vi "FeedbackDecode_BuildMSMSSphere.vi"(4 "CompArray":T2(array[cluster])=[{"Name"="\"LittleSphereJ\"", "Type"="\"Trans3Joint\"", "ID"="J", "Num"="86", "COM"=[], "Offset"=[], "RotationAxis"=[], "OrientationMatrix"=[[1.0, 0.0, 0.0], [0.0, 1.0, 0.0], [0.0, 0.0, 1.0]], "MinAngle"=nan, "MaxAngle"=nan, "InboardID"="S", "InboardNum"="1110", "InboardCOM"=[0.0, 0.0, 0.0], "OutboardID"="S", "OutboardNum"="84", "OutboardCOM"=[0.0, 0.0, 0.0]}, {"Name"="\"IndexSphereJ\"", "Type"="\"Trans3Joint\"", "ID"="J", "Num"="94", "COM"=[], "Offset"=[], "RotationAxis"=[], "OrientationMatrix"=[[1.0, 0.0, 0.0], [0.0, 1.0, 0.0], [0.0, 0.0, 1.0]], "MinAngle"=nan, "MaxAngle"=nan, "InboardID"="S", "InboardNum"="1110", "InboardCOM"=[0.0, 0.0, 0.0], "OutboardID"="S", "OutboardNum"="92", "OutboardCOM"=[0.0, 0.0, 0.0]}, {"Name"="\"LittleKnuckle\"", "Type"="\"PinJoint\"", "ID"="J", "Num"="1160", "COM"=[], "Offset"=[], "RotationAxis"=[-0.982409, 0.0686967, 0.173648], "OrientationMatrix"=[[1.0, 0.0, 0.0], [0.0, 1.0, 0.0], [0.0, 0.0, 1.0]], "MinAngle"=0.0, "MaxAngle"=3.140021857262998, "InboardID"="S", "InboardNum"="1122", "InboardCOM"=[-0.01026417, -0.01431899999999997, 0.005183300000000002], "OutboardID"="S", "OutboardNum"="112", "OutboardCOM"=[0.0, 0.0, 0.0]}, {"Name"="\"LittleSide\"", "Type"="\"PinJoint\"", "ID"="J", "Num"="1161", "COM"=[], "Offset"=[], "RotationAxis"=[0.173225, -0.0121131, -0.984808], "OrientationMatrix"=[[1.0, 0.0, 0.0], [0.0, 1.0, 0.0], [0.0, 0.0, 1.0]], "MinAngle"=0.0, "MaxAngle"=3.140021857262998, "InboardID"="S", "InboardNum"="1110", "InboardCOM"=[-0.02813713, -0.080592, -0.0049779], "OutboardID"="S", "OutboardNum"="1122", "OutboardCOM"=[0.0, 0.0, 0.0]}, {"Name"="\"RingPIP\"", "Type"="\"PinJoint\"", "ID"="J", "Num"="1162", "COM"=[], "Offset"=[], "RotationAxis"=[-0.993768, 0.069491, 0.0871557], "OrientationMatrix"=[[1.0, 0.0, 0.0], [0.0, 1.0, 0.0], [0.0, 0.0, 1.0]], "MinAngle"=0.0, "MaxAngle"=3.140021857262998, "InboardID"="S", "InboardNum"="1125", "InboardCOM"=[-0.00263497, -0.03339700000000001, 2.619999999999706e-05], "OutboardID"="S", "OutboardNum"="1121", "OutboardCOM"=[0.0, 0.0, 0.0]}, {"Name"="\"ThumbKnuckle\"", "Type"="\"PinJoint\"", "ID"="J", "Num"="1163", "COM"=[], "Offset"=[], "RotationAxis"=[-0.130028, -0.197163, -0.97171], "OrientationMatrix"=[[1.0, 0.0, 0.0], [0.0, 1.0, 0.0], [0.0, 0.0, 1.0]], "MinAngle"=0.0, "MaxAngle"=3.140021857262998, "InboardID"="S", "InboardNum"="1113", "InboardCOM"=[0.0221366, -0.0038129999999999553, 0.00214783], "OutboardID"="S", "OutboardNum"="111", "OutboardCOM"=[0.0, 0.0, 0.0]}, {"Name"="\"RingSide\"", "Type"="\"PinJoint\"", "ID"="J", "Num"="1164", "COM"=[], "Offset"=[], "RotationAxis"=[0.0869434, -0.00607968, -0.996195], "OrientationMatrix"=[[1.0, 0.0, 0.0], [0.0, 1.0, 0.0], [0.0, 0.0, 1.0]], "MinAngle"=0.0, "MaxAngle"=3.140021857262998, "InboardID"="S", "InboardNum"="1110", "InboardCOM"=[-0.0087988, -0.08356699999999995, -0.008058199999999998], "OutboardID"="S", "OutboardNum"="1123", "OutboardCOM"=[0.0, 0.0, 0.0]}, {"Name"="\"RingKnuckle\"", "Type"="\"PinJoint\"", "ID"="J", "Num"="1165", "COM"=[], "Offset"=[], "RotationAxis"=[-0.993768, 0.069491, 0.0871557], "OrientationMatrix"=[[1.0, 0.0, 0.0], [0.0, 1.0, 0.0], [0.0, 0.0, 1.0]], "MinAngle"=0.0, "MaxAngle"=3.140021857262998, "InboardID"="S", "InboardNum"="1123", "InboardCOM"=[-0.01067969, -0.014290000000000025, 0.0043582], "OutboardID"="S", "OutboardNum"="1125", "OutboardCOM"=[0.0, 0.0, 0.0]}, {"Name"="\"ShoulderRoll\"", "Type"="\"PinJoint\"", "ID"="J", "Num"="1166", "COM"=[], "Offset"=[], "RotationAxis"=[0.0, -1.0, 0.0], "OrientationMatrix"=[[1.0, 0.0, 0.0], [0.0, 1.0, 0.0], [0.0, 0.0, 1.0]], "MinAngle"=0.0, "MaxAngle"=3.140021857262998, "InboardID"="S", "InboardNum"="1127", "InboardCOM"=[0.0346, -0.26093099999999997, 0.0], "OutboardID"="S", "OutboardNum"="116", "OutboardCOM"=[0.0, 0.0, 0.0]}, {"Name"="\"MiddleDIP\"", "Type"="\"PinJoint\"", "ID"="J", "Num"="1167", "COM"=[], "Offset"=[], "RotationAxis"=[-1.0, 0.0, 0.0], "OrientationMatrix"=[[1.0, 0.0, 0.0], [0.0, 1.0, 0.0], [0.0, 0.0, 1.0]], "MinAngle"=0.0, "MaxAngle"=3.14, "InboardID"="S", "InboardNum"="113", "InboardCOM"=[0.0197, -0.022077000000000013, -0.0010000000000000009], "OutboardID"="S", "OutboardNum"="1114", "OutboardCOM"=[0.0, 0.0, 0.0]}, {"Name"="\"IndexDIP\"", "Type"="\"PinJoint\"", "ID"="J", "Num"="1168", "COM"=[], "Offset"=[], "RotationAxis"=[-1.0, 0.0, 0.0], "OrientationMatrix"=[[1.0, 0.0, 0.0], [0.0, 1.0, 0.0], [0.0, 0.0, 1.0]], "MinAngle"=0.0, "MaxAngle"=3.140021857262998, "InboardID"="S", "InboardNum"="1124", "InboardCOM"=[0.019699999999999995, -0.017971999999999988, -0.0009999999999999974], "OutboardID"="S", "OutboardNum"="1117", "OutboardCOM"=[0.0, 0.0, 0.0]}, {"Name"="\"IndexKnuckle\"", "Type"="\"PinJoint\"", "ID"="J", "Num"="1169", "COM"=[], "Offset"=[], "RotationAxis"=[-1.0, 0.0, 0.0], "OrientationMatrix"=[[1.0, 0.0, 0.0], [0.0, 1.0, 0.0], [0.0, 0.0, 1.0]], "MinAngle"=0.0, "MaxAngle"=3.140021857262998, "InboardID"="S", "InboardNum"="1118", "InboardCOM"=[-0.0071716, -0.017827999999999955, 0.0025407999999999993], "OutboardID"="S", "OutboardNum"="1126", "OutboardCOM"=[0.0, 0.0, 0.0]}, {"Name"="\"MiddleKnuckle\"", "Type"="\"PinJoint\"", "ID"="J", "Num"="1170", "COM"=[], "Offset"=[], "RotationAxis"=[-1.0, 0.0, 0.0], "OrientationMatrix"=[[1.0, 0.0, 0.0], [0.0, 1.0, 0.0], [0.0, 0.0, 1.0]], "MinAngle"=0.0, "MaxAngle"=3.140021857262998, "InboardID"="S", "InboardNum"="1110", "InboardCOM"=[-0.00031180000000000097, -0.09855000000000003, -0.0048641], "OutboardID"="S", "OutboardNum"="1119", "OutboardCOM"=[0.0, 0.0, 0.0]}, {"Name"="\"RingSphereJ\"", "Type"="\"Trans3Joint\"", "ID"="J", "Num"="15", "COM"=[], "Offset"=[], "RotationAxis"=[], "OrientationMatrix"=[[1.0, 0.0, 0.0], [0.0, 1.0, 0.0], [0.0, 0.0, 1.0]], "MinAngle"=nan, "MaxAngle"=nan, "InboardID"="S", "InboardNum"="1110", "InboardCOM"=[0.0, 0.0, 0.0], "OutboardID"="S", "OutboardNum"="18", "OutboardCOM"=[0.0, 0.0, 0.0]}, {"Name"="\"MiddleSphereJ\"", "Type"="\"Trans3Joint\"", "ID"="J", "Num"="11", "COM"=[], "Offset"=[], "RotationAxis"=[], "OrientationMatrix"=[[1.0, 0.0, 0.0], [0.0, 1.0, 0.0], [0.0, 0.0, 1.0]], "MinAngle"=nan, "MaxAngle"=nan, "InboardID"="S", "InboardNum"="1110", "InboardCOM"=[0.0, 0.0, 0.0], "OutboardID"="S", "OutboardNum"="14", "OutboardCOM"=[0.0, 0.0, 0.0]}, {"Name"="\"ThumbSphereJ\"", "Type"="\"Trans3Joint\"", "ID"="J", "Num"="23", "COM"=[], "Offset"=[], "RotationAxis"=[], "OrientationMatrix"=[[1.0, 0.0, 0.0], [0.0, 1.0, 0.0], [0.0, 0.0, 1.0]], "MinAngle"=nan, "MaxAngle"=nan, "InboardID"="S", "InboardNum"="1110", "InboardCOM"=[0.0, 0.0, 0.0], "OutboardID"="S", "OutboardNum"="22", "OutboardCOM"=[0.0, 0.0, 0.0]}, {"Name"="\"RingDIP\"", "Type"="\"PinJoint\"", "ID"="J", "Num"="1144", "COM"=[], "Offset"=[], "RotationAxis"=[-0.993768, 0.069491, 0.0871557], "OrientationMatrix"=[[1.0, 0.0, 0.0], [0.0, 1.0, 0.0], [0.0, 0.0, 1.0]], "MinAngle"=0.0, "MaxAngle"=3.140021857262998, "InboardID"="S", "InboardNum"="1121", "InboardCOM"=[0.01818386, -0.020046000000000008, -0.002713199999999999], "OutboardID"="S", "OutboardNum"="115", "OutboardCOM"=[0.0, 0.0, 0.0]}, {"Name"="\"ElbowPitch\"", "Type"="\"PinJoint\"", "ID"="J", "Num"="1145", "COM"=[], "Offset"=[], "RotationAxis"=[0.0, 0.0, 1.0], "OrientationMatrix"=[[1.0, 0.0, 0.0], [0.0, 1.0, 0.0], [0.0, 0.0, 1.0]], "MinAngle"=0.0, "MaxAngle"=3.140021857262998, "InboardID"="S", "InboardNum"="116", "InboardCOM"=[0.019, -0.013836000000000015, -0.009000000000000001], "OutboardID"="S", "OutboardNum"="1111", "OutboardCOM"=[0.0, 0.0, 0.0]}, {"Name"="\"WristPitch\"", "Type"="\"PinJoint\"", "ID"="J", "Num"="1146", "COM"=[], "Offset"=[], "RotationAxis"=[-1.0, 0.0, 0.0], "OrientationMatrix"=[[1.0, 0.0, 0.0], [0.0, 1.0, 0.0], [0.0, 0.0, 1.0]], "MinAngle"=-0.7853981633974483, "MaxAngle"=0.7853981633974483, "InboardID"="S", "InboardNum"="114", "InboardCOM"=[0.042499999999999996, -0.16914000000000007, 0.0], "OutboardID"="S", "OutboardNum"="119", "OutboardCOM"=[0.0, 0.0, 0.0]}, {"Name"="\"ThumbDIP\"", "Type"="\"PinJoint\"", "ID"="J", "Num"="1147", "COM"=[], "Offset"=[], "RotationAxis"=[-0.130028, -0.197163, -0.97171], "OrientationMatrix"=[[1.0, 0.0, 0.0], [0.0, 1.0, 0.0], [0.0, 0.0, 1.0]], "MinAngle"=0.0, "MaxAngle"=3.14, "InboardID"="S", "InboardNum"="111", "InboardCOM"=[0.018637, -0.022448000000000023, -0.01061123], "OutboardID"="S", "OutboardNum"="1116", "OutboardCOM"=[0.0, 0.0, 0.0]}, {"Name"="\"IndexSide\"", "Type"="\"PinJoint\"", "ID"="J", "Num"="1148", "COM"=[], "Offset"=[], "RotationAxis"=[0.0, 0.0, -1.0], "OrientationMatrix"=[[1.0, 0.0, 0.0], [0.0, 1.0, 0.0], [0.0, 0.0, 1.0]], "MinAngle"=0.0, "MaxAngle"=3.140021857262998, "InboardID"="S", "InboardNum"="1110", "InboardCOM"=[0.027229700000000003, -0.07779400000000003, -0.0051141], "OutboardID"="S", "OutboardNum"="1118", "OutboardCOM"=[0.0, 0.0, 0.0]}, {"Name"="\"MiddlePIP\"", "Type"="\"PinJoint\"", "ID"="J", "Num"="1149", "COM"=[], "Offset"=[], "RotationAxis"=[-1.0, 0.0, 0.0], "OrientationMatrix"=[[1.0, 0.0, 0.0], [0.0, 1.0, 0.0], [0.0, 0.0, 1.0]], "MinAngle"=0.0, "MaxAngle"=3.140021857262998, "InboardID"="S", "InboardNum"="1119", "InboardCOM"=[-0.0002999999999999982, -0.0383, 0.0], "OutboardID"="S", "OutboardNum"="113", "OutboardCOM"=[0.0, 0.0, 0.0]}, {"Name"="\"ShoulderYaw\"", "Type"="\"PinJoint\"", "ID"="J", "Num"="1150", "COM"=[], "Offset"=[], "RotationAxis"=[0.0, 0.0, 1.0], "OrientationMatrix"=[[1.0, 0.0, 0.0], [0.0, 1.0, 0.0], [0.0, 0.0, 1.0]], "MinAngle"=0.0, "MaxAngle"=3.140021857262998, "InboardID"="S", "InboardNum"="117", "InboardCOM"=[-1.45121e-10, 0.000384746, -0.003098433], "OutboardID"="S", "OutboardNum"="1120", "OutboardCOM"=[0.0, 0.0, 0.0]}, {"Name"="\"ThumbSide\"", "Type"="\"PinJoint\"", "ID"="J", "Num"="1151", "COM"=[], "Offset"=[], "RotationAxis"=[0.691978, 0.683845, -0.23135], "OrientationMatrix"=[[1.0, 0.0, 0.0], [0.0, 1.0, 0.0], [0.0, 0.0, 1.0]], "MinAngle"=-0.7853981633974483, "MaxAngle"=0.7853981633974483, "InboardID"="S", "InboardNum"="118", "InboardCOM"=[0.008416800000000002, -0.028861000000000026, 0.0017169000000000004], "OutboardID"="S", "OutboardNum"="1113", "OutboardCOM"=[0.0, 0.0, 0.0]}, {"Name"="\"LittleDIP\"", "Type"="\"PinJoint\"", "ID"="J", "Num"="1152", "COM"=[], "Offset"=[], "RotationAxis"=[-0.982409, 0.0686967, 0.173648], "OrientationMatrix"=[[1.0, 0.0, 0.0], [0.0, 1.0, 0.0], [0.0, 0.0, 1.0]], "MinAngle"=0.0, "MaxAngle"=3.140021857262998, "InboardID"="S", "InboardNum"="1115", "InboardCOM"=[0.01887955, -0.014112000000000013, -0.004509900000000001], "OutboardID"="S", "OutboardNum"="1112", "OutboardCOM"=[0.0, 0.0, 0.0]}, {"Name"="\"WristYaw\"", "Type"="\"PinJoint\"", "ID"="J", "Num"="1153", "COM"=[], "Offset"=[], "RotationAxis"=[0.0, 0.0, -1.0], "OrientationMatrix"=[[1.0, 0.0, 0.0], [0.0, 1.0, 0.0], [0.0, 0.0, 1.0]], "MinAngle"=-0.7853981633974483, "MaxAngle"=0.7853981633974483, "InboardID"="S", "InboardNum"="119", "InboardCOM"=[-0.0425218, -0.006901999999999964, -0.004796100000000001], "OutboardID"="S", "OutboardNum"="1110", "OutboardCOM"=[0.0, 0.0, 0.0]}, {"Name"="\"IndexPIP\"", "Type"="\"PinJoint\"", "ID"="J", "Num"="1154", "COM"=[], "Offset"=[], "RotationAxis"=[-1.0, 0.0, 0.0], "OrientationMatrix"=[[1.0, 0.0, 0.0], [0.0, 1.0, 0.0], [0.0, 0.0, 1.0]], "MinAngle"=0.0, "MaxAngle"=3.140021857262998, "InboardID"="S", "InboardNum"="1126", "InboardCOM"=[-0.00030000000000000165, -0.03400000000000003, 0.0], "OutboardID"="S", "OutboardNum"="1124", "OutboardCOM"=[0.0, 0.0, 0.0]}, {"Name"="\"LittlePIP\"", "Type"="\"PinJoint\"", "ID"="J", "Num"="1155", "COM"=[], "Offset"=[], "RotationAxis"=[-0.982409, 0.0686967, 0.173648], "OrientationMatrix"=[[1.0, 0.0, 0.0], [0.0, 1.0, 0.0], [0.0, 0.0, 1.0]], "MinAngle"=0.0, "MaxAngle"=3.140021857262998, "InboardID"="S", "InboardNum"="112", "InboardCOM"=[-0.0021084, -0.02591600000000005, 5.209999999999937e-05], "OutboardID"="S", "OutboardNum"="1115", "OutboardCOM"=[0.0, 0.0, 0.0]}, {"Name"="\"ThumbMeta\"", "Type"="\"PinJoint\"", "ID"="J", "Num"="1156", "COM"=[], "Offset"=[], "RotationAxis"=[-0.0212682, -0.997909, -0.0610298], "OrientationMatrix"=[[1.0, 0.0, 0.0], [0.0, 1.0, 0.0], [0.0, 0.0, 1.0]], "MinAngle"=0.0, "MaxAngle"=3.14, "InboardID"="S", "InboardNum"="1110", "InboardCOM"=[0.015011799999999999, -0.011859999999999982, 0.0126182], "OutboardID"="S", "OutboardNum"="118", "OutboardCOM"=[0.0, 0.0, 0.0]}, {"Name"="\"ShoulderOblique\"", "Type"="\"PinJoint\"", "ID"="J", "Num"="1157", "COM"=[], "Offset"=[], "RotationAxis"=[0.57735, 0.57735, 0.57735], "OrientationMatrix"=[[1.0, 0.0, 0.0], [0.0, 1.0, 0.0], [0.0, 0.0, 1.0]], "MinAngle"=0.0, "MaxAngle"=3.14, "InboardID"="S", "InboardNum"="12", "InboardCOM"=[-0.09, -0.05, -0.26], "OutboardID"="S", "OutboardNum"="117", "OutboardCOM"=[0.0, 0.0, 0.0]}, {"Name"="\"ShoulderPitch\"", "Type"="\"PinJoint\"", "ID"="J", "Num"="1158", "COM"=[], "Offset"=[], "RotationAxis"=[-1.0, 0.0, 0.0], "OrientationMatrix"=[[1.0, 0.0, 0.0], [0.0, 1.0, 0.0], [0.0, 0.0, 1.0]], "MinAngle"=0.0, "MaxAngle"=3.140021857262998, "InboardID"="S", "InboardNum"="1120", "InboardCOM"=[-0.0346, -0.005, -0.0125], "OutboardID"="S", "OutboardNum"="1127", "OutboardCOM"=[0.0, 0.0, 0.0]}, {"Name"="\"WristRoll\"", "Type"="\"PinJoint\"", "ID"="J", "Num"="1159", "COM"=[], "Offset"=[], "RotationAxis"=[0.0, -1.0, 0.0], "OrientationMatrix"=[[1.0, 0.0, 0.0], [0.0, 1.0, 0.0], [0.0, 0.0, 1.0]], "MinAngle"=-1.5707963267948966, "MaxAngle"=1.5707963267948966, "InboardID"="S", "InboardNum"="1111", "InboardCOM"=[0.0, -0.06298999999999999, 0.003020000000000002], "OutboardID"="S", "OutboardNum"="114", "OutboardCOM"=[0.0, 0.0, 0.0]}, {"Name"="\"WristSphereJ\"", "Type"="\"Trans3Joint\"", "ID"="J", "Num"="88", "COM"=[], "Offset"=[], "RotationAxis"=[], "OrientationMatrix"=[[1.0, 0.0, 0.0], [0.0, 1.0, 0.0], [0.0, 0.0, 1.0]], "MinAngle"=nan, "MaxAngle"=nan, "InboardID"="S", "InboardNum"="114", "InboardCOM"=[0.0, 0.0, 0.0], "OutboardID"="S", "OutboardNum"="87", "OutboardCOM"=[0.0, 0.0, 0.0]}, {"Name"="\"LittleSphere\"", "Type"="\"Segment\"", "ID"="S", "Num"="84", "COM"=[0.0, 0.0, 0.0], "Offset"=[0.0, 0.0, 0.0], "RotationAxis"=[], "OrientationMatrix"=[], "MinAngle"=nan, "MaxAngle"=nan, "InboardID"="", "InboardNum"="", "InboardCOM"=[], "OutboardID"="", "OutboardNum"="", "OutboardCOM"=[]}, {"Name"="\"IndexSphere\"", "Type"="\"Segment\"", "ID"="S", "Num"="92", "COM"=[0.0, 0.0, 0.0], "Offset"=[0.0, 0.0, 0.0], "RotationAxis"=[], "OrientationMatrix"=[], "MinAngle"=nan, "MaxAngle"=nan, "InboardID"="", "InboardNum"="", "InboardCOM"=[], "OutboardID"="", "OutboardNum"="", "OutboardCOM"=[]}, {"Name"="\"ShoulderHR\"", "Type"="\"Segment\"", "ID"="S", "Num"="1127", "COM"=[0.03942751, -0.096221, -2.3999999999996247e-06], "Offset"=[0.0346, 0.005, 0.01541], "RotationAxis"=[], "OrientationMatrix"=[], "MinAngle"=nan, "MaxAngle"=nan, "InboardID"="", "InboardNum"="", "InboardCOM"=[], "OutboardID"="", "OutboardNum"="", "OutboardCOM"=[]}, {"Name"="\"ThumbProximal\"", "Type"="\"Segment\"", "ID"="S", "Num"="111", "COM"=[0.010053400000000004, -0.01129800000000003, -0.003517029999999999], "Offset"=[-0.0645434, 0.563333, 0.00970317], "RotationAxis"=[], "OrientationMatrix"=[], "MinAngle"=nan, "MaxAngle"=nan, "InboardID"="", "InboardNum"="", "InboardCOM"=[], "OutboardID"="", "OutboardNum"="", "OutboardCOM"=[]}, {"Name"="\"LittleProximal\"", "Type"="\"Segment\"", "ID"="S", "Num"="112", "COM"=[0.0086144, -0.013174000000000019, -0.0019825000000000016], "Offset"=[0.0194231, 0.61371, 0.0259807], "RotationAxis"=[], "OrientationMatrix"=[], "MinAngle"=nan, "MaxAngle"=nan, "InboardID"="", "InboardNum"="", "InboardCOM"=[], "OutboardID"="", "OutboardNum"="", "OutboardCOM"=[]}, {"Name"="\"MiddleMedial\"", "Type"="\"Segment\"", "ID"="S", "Num"="113", "COM"=[0.009050299999999997, -0.011116000000000015, -0.0009771999999999975], "Offset"=[-0.0183664, 0.655649, 0.0310502], "RotationAxis"=[], "OrientationMatrix"=[], "MinAngle"=nan, "MaxAngle"=nan, "InboardID"="", "InboardNum"="", "InboardCOM"=[], "OutboardID"="", "OutboardNum"="", "OutboardCOM"=[]}, {"Name"="\"Forearm\"", "Type"="\"Segment\"", "ID"="S", "Num"="114", "COM"=[-1.860000000000056e-05, -0.08232500000000004, -9.750000000000036e-05], "Offset"=[-0.019, 0.342757, 0.02139], "RotationAxis"=[], "OrientationMatrix"=[], "MinAngle"=nan, "MaxAngle"=nan, "InboardID"="", "InboardNum"="", "InboardCOM"=[], "OutboardID"="", "OutboardNum"="", "OutboardCOM"=[]}, {"Name"="\"RingDistal\"", "Type"="\"Segment\"", "ID"="S", "Num"="115", "COM"=[-0.01039068, -0.008301000000000003, 0.0005073999999999981], "Offset"=[-0.0150486, 0.670099, 0.0325731], "RotationAxis"=[], "OrientationMatrix"=[], "MinAngle"=nan, "MaxAngle"=nan, "InboardID"="", "InboardNum"="", "InboardCOM"=[], "OutboardID"="", "OutboardNum"="", "OutboardCOM"=[]}, {"Name"="\"HR TO ELBOW_1\"", "Type"="\"Segment\"", "ID"="S", "Num"="116", "COM"=[0.0103972, 0.026906999999999986, 0.0011380000000000001], "Offset"=[0.0, 0.265931, 0.01541], "RotationAxis"=[], "OrientationMatrix"=[], "MinAngle"=nan, "MaxAngle"=nan, "InboardID"="", "InboardNum"="", "InboardCOM"=[], "OutboardID"="", "OutboardNum"="", "OutboardCOM"=[]}, {"Name"="\"ShoulderSocket\"", "Type"="\"Segment\"", "ID"="S", "Num"="117", "COM"=[0.0, 0.0, 0.0], "Offset"=[-1.45121e-10, 0.000384746, -0.000188433], "RotationAxis"=[], "OrientationMatrix"=[], "MinAngle"=nan, "MaxAngle"=nan, "InboardID"="", "InboardNum"="", "InboardCOM"=[], "OutboardID"="", "OutboardNum"="", "OutboardCOM"=[]}, {"Name"="\"ThumbRoll\"", "Type"="\"Segment\"", "ID"="S", "Num"="118", "COM"=[0.005574799999999998, -0.01721499999999998, -0.0012329999999999997], "Offset"=[-0.03399, 0.530659, 0.0135679], "RotationAxis"=[], "OrientationMatrix"=[], "MinAngle"=nan, "MaxAngle"=nan, "InboardID"="", "InboardNum"="", "InboardCOM"=[], "OutboardID"="", "OutboardNum"="", "OutboardCOM"=[]}, {"Name"="\"WristFlex\"", "Type"="\"Segment\"", "ID"="S", "Num"="119", "COM"=[-0.0420033, -0.003865999999999925, 0.000690699999999999], "Offset"=[-0.0615, 0.511897, 0.02139], "RotationAxis"=[], "OrientationMatrix"=[], "MinAngle"=nan, "MaxAngle"=nan, "InboardID"="", "InboardNum"="", "InboardCOM"=[], "OutboardID"="", "OutboardNum"="", "OutboardCOM"=[]}, {"Name"="\"ThumbSphere\"", "Type"="\"Segment\"", "ID"="S", "Num"="22", "COM"=[0.0, 0.0, 0.0], "Offset"=[0.0, 0.0, 0.0], "RotationAxis"=[], "OrientationMatrix"=[], "MinAngle"=nan, "MaxAngle"=nan, "InboardID"="", "InboardNum"="", "InboardCOM"=[], "OutboardID"="", "OutboardNum"="", "OutboardCOM"=[]}, {"Name"="\"RingSphere\"", "Type"="\"Segment\"", "ID"="S", "Num"="18", "COM"=[0.0, 0.0, 0.0], "Offset"=[0.0, 0.0, 0.0], "RotationAxis"=[], "OrientationMatrix"=[], "MinAngle"=nan, "MaxAngle"=nan, "InboardID"="", "InboardNum"="", "InboardCOM"=[], "OutboardID"="", "OutboardNum"="", "OutboardCOM"=[]}, {"Name"="\"MiddleSphere\"", "Type"="\"Segment\"", "ID"="S", "Num"="14", "COM"=[0.0, 0.0, 0.0], "Offset"=[0.0, 0.0, 0.0], "RotationAxis"=[], "OrientationMatrix"=[], "MinAngle"=nan, "MaxAngle"=nan, "InboardID"="", "InboardNum"="", "InboardCOM"=[], "OutboardID"="", "OutboardNum"="", "OutboardCOM"=[]}, {"Name"="\"PalmAssembly\"", "Type"="\"Segment\"", "ID"="S", "Num"="1110", "COM"=[5.000000000005e-07, -0.049819999999999975, 0.0028357999999999994], "Offset"=[-0.0189782, 0.518799, 0.0261861], "RotationAxis"=[], "OrientationMatrix"=[], "MinAngle"=nan, "MaxAngle"=nan, "InboardID"="", "InboardNum"="", "InboardCOM"=[], "OutboardID"="", "OutboardNum"="", "OutboardCOM"=[]}, {"Name"="\"ELBOW TO RR_1\"", "Type"="\"Segment\"", "ID"="S", "Num"="1111", "COM"=[-0.0009622999999999993, -0.06578500000000004, 0.0023389000000000014], "Offset"=[-0.019, 0.279767, 0.02441], "RotationAxis"=[], "OrientationMatrix"=[], "MinAngle"=nan, "MaxAngle"=nan, "InboardID"="", "InboardNum"="", "InboardCOM"=[], "OutboardID"="", "OutboardNum"="", "OutboardCOM"=[]}, {"Name"="\"LittleDistal\"", "Type"="\"Segment\"", "ID"="S", "Num"="1112", "COM"=[-0.01022215, -0.006736999999999993, 0.0015411999999999995], "Offset"=[0.00265195, 0.653738, 0.0304385], "RotationAxis"=[], "OrientationMatrix"=[], "MinAngle"=nan, "MaxAngle"=nan, "InboardID"="", "InboardNum"="", "InboardCOM"=[], "OutboardID"="", "OutboardNum"="", "OutboardCOM"=[]}, {"Name"="\"ThumbMedial\"", "Type"="\"Segment\"", "ID"="S", "Num"="1113", "COM"=[0.014731999999999995, 0.003503000000000034, -0.0037245000000000004], "Offset"=[-0.0424068, 0.55952, 0.011851], "RotationAxis"=[], "OrientationMatrix"=[], "MinAngle"=nan, "MaxAngle"=nan, "InboardID"="", "InboardNum"="", "InboardCOM"=[], "OutboardID"="", "OutboardNum"="", "OutboardCOM"=[]}, {"Name"="\"MiddleDistal\"", "Type"="\"Segment\"", "ID"="S", "Num"="1114", "COM"=[-0.0100904, -0.008909999999999973, -0.00043409999999999976], "Offset"=[-0.0380664, 0.677726, 0.0320502], "RotationAxis"=[], "OrientationMatrix"=[], "MinAngle"=nan, "MaxAngle"=nan, "InboardID"="", "InboardNum"="", "InboardCOM"=[], "OutboardID"="", "OutboardNum"="", "OutboardCOM"=[]}, {"Name"="\"LittleMedial\"", "Type"="\"Segment\"", "ID"="S", "Num"="1115", "COM"=[0.009976699999999998, -0.005878999999999968, -0.002634000000000001], "Offset"=[0.0215315, 0.639626, 0.0259286], "RotationAxis"=[], "OrientationMatrix"=[], "MinAngle"=nan, "MaxAngle"=nan, "InboardID"="", "InboardNum"="", "InboardCOM"=[], "OutboardID"="", "OutboardNum"="", "OutboardCOM"=[]}, {"Name"="\"ThumbDistal\"", "Type"="\"Segment\"", "ID"="S", "Num"="1116", "COM"=[0.0094852, -0.005989000000000022, 0.008354], "Offset"=[-0.0831804, 0.585781, 0.0203144], "RotationAxis"=[], "OrientationMatrix"=[], "MinAngle"=nan, "MaxAngle"=nan, "InboardID"="", "InboardNum"="", "InboardCOM"=[], "OutboardID"="", "OutboardNum"="", "OutboardCOM"=[]}, {"Name"="\"IndexDistal\"", "Type"="\"Segment\"", "ID"="S", "Num"="1117", "COM"=[-0.009959199999999994, -0.007608999999999977, -6.570000000000187e-05], "Offset"=[-0.0584363, 0.666393, 0.0297594], "RotationAxis"=[], "OrientationMatrix"=[], "MinAngle"=nan, "MaxAngle"=nan, "InboardID"="", "InboardNum"="", "InboardCOM"=[], "OutboardID"="", "OutboardNum"="", "OutboardCOM"=[]}, {"Name"="\"MCPIndex\"", "Type"="\"Segment\"", "ID"="S", "Num"="1118", "COM"=[0.0017073999999999978, -0.006472999999999951, 0.002308899999999999], "Offset"=[-0.0462079, 0.596593, 0.0313002], "RotationAxis"=[], "OrientationMatrix"=[], "MinAngle"=nan, "MaxAngle"=nan, "InboardID"="", "InboardNum"="", "InboardCOM"=[], "OutboardID"="", "OutboardNum"="", "OutboardCOM"=[]}, {"Name"="\"MiddleProximal\"", "Type"="\"Segment\"", "ID"="S", "Num"="1119", "COM"=[0.009659500000000001, -0.017927999999999944, -8.019999999999902e-05], "Offset"=[-0.0186664, 0.617349, 0.0310502], "RotationAxis"=[], "OrientationMatrix"=[], "MinAngle"=nan, "MaxAngle"=nan, "InboardID"="", "InboardNum"="", "InboardCOM"=[], "OutboardID"="", "OutboardNum"="", "OutboardCOM"=[]}, {"Name"="\"ShoulderGearMotor\"", "Type"="\"Segment\"", "ID"="S", "Num"="1120", "COM"=[0.0067537, -0.00104092, -0.0093986], "Offset"=[0.0, 0.0, 0.00291], "RotationAxis"=[], "OrientationMatrix"=[], "MinAngle"=nan, "MaxAngle"=nan, "InboardID"="", "InboardNum"="", "InboardCOM"=[], "OutboardID"="", "OutboardNum"="", "OutboardCOM"=[]}, {"Name"="\"RingMedial\"", "Type"="\"Segment\"", "ID"="S", "Num"="1121", "COM"=[0.00875476, -0.00992700000000002, -0.0017671999999999966], "Offset"=[0.00313526, 0.650053, 0.0298599], "RotationAxis"=[], "OrientationMatrix"=[], "MinAngle"=nan, "MaxAngle"=nan, "InboardID"="", "InboardNum"="", "InboardCOM"=[], "OutboardID"="", "OutboardNum"="", "OutboardCOM"=[]}, {"Name"="\"MCPLittle\"", "Type"="\"Segment\"", "ID"="S", "Num"="1122", "COM"=[4.4959999999998404e-05, -0.007433999999999941, 0.0037990000000000003], "Offset"=[0.00915893, 0.599391, 0.031164], "RotationAxis"=[], "OrientationMatrix"=[], "MinAngle"=nan, "MaxAngle"=nan, "InboardID"="", "InboardNum"="", "InboardCOM"=[], "OutboardID"="", "OutboardNum"="", "OutboardCOM"=[]}, {"Name"="\"MCPRing\"", "Type"="\"Segment\"", "ID"="S", "Num"="1123", "COM"=[0.00014349999999999953, -0.007109000000000032, 0.003743], "Offset"=[-0.0101794, 0.602366, 0.0342443], "RotationAxis"=[], "OrientationMatrix"=[], "MinAngle"=nan, "MaxAngle"=nan, "InboardID"="", "InboardNum"="", "InboardCOM"=[], "OutboardID"="", "OutboardNum"="", "OutboardCOM"=[]}, {"Name"="\"IndexMedial\"", "Type"="\"Segment\"", "ID"="S", "Num"="1124", "COM"=[0.009597399999999999, -0.008967999999999976, -0.0012315999999999994], "Offset"=[-0.0387363, 0.648421, 0.0287594], "RotationAxis"=[], "OrientationMatrix"=[], "MinAngle"=nan, "MaxAngle"=nan, "InboardID"="", "InboardNum"="", "InboardCOM"=[], "OutboardID"="", "OutboardNum"="", "OutboardCOM"=[]}, {"Name"="\"RingProximal\"", "Type"="\"Segment\"", "ID"="S", "Num"="1125", "COM"=[0.008387790000000001, -0.01778599999999997, -0.0011962000000000014], "Offset"=[0.00050029, 0.616656, 0.0298861], "RotationAxis"=[], "OrientationMatrix"=[], "MinAngle"=nan, "MaxAngle"=nan, "InboardID"="", "InboardNum"="", "InboardCOM"=[], "OutboardID"="", "OutboardNum"="", "OutboardCOM"=[]}, {"Name"="\"IndexProximal\"", "Type"="\"Segment\"", "ID"="S", "Num"="1126", "COM"=[0.010082999999999995, -0.01634599999999997, -0.00038749999999999896], "Offset"=[-0.0390363, 0.614421, 0.0287594], "RotationAxis"=[], "OrientationMatrix"=[], "MinAngle"=nan, "MaxAngle"=nan, "InboardID"="", "InboardNum"="", "InboardCOM"=[], "OutboardID"="", "OutboardNum"="", "OutboardCOM"=[]}, {"Name"="\"WristSphere\"", "Type"="\"Segment\"", "ID"="S", "Num"="87", "COM"=[0.0, 0.0, 0.0], "Offset"=[0.0, 0.0, 0.0], "RotationAxis"=[], "OrientationMatrix"=[], "MinAngle"=nan, "MaxAngle"=nan, "InboardID"="", "InboardNum"="", "InboardCOM"=[], "OutboardID"="", "OutboardNum"="", "OutboardCOM"=[]}], 6 "ModelParams":T1={"ModelName"="MaleLeft4\nMaleLeft4", "Value"=[[0.002, -0.01, 0.0015], [0.0, 45.0, 0.0], [-40.0, 40.0, 0.0], [0.0, 50.0, 0.0], [0.0, 75.0, 0.0], [0.0, -0.007, 0.005], [10.0, -13.0, 0.0], [0.0, 75.0, 0.0], [0.0, 75.0, 0.0], [0.0, 45.0, 0.0], [0.0, -0.005, 0.0055], [0.0, 75.0, 0.0], [0.0, 75.0, 0.0], [0.0, 45.0, 0.0], [0.0, -0.005, 0.0045], [-10.0, 10.0, 0.0], [0.0, 75.0, 0.0], [0.0, 75.0, 0.0], [0.0, 45.0, 0.0], [0.0006, -0.005, 0.0045], [-8.0, 15.0, 0.0], [0.0, 75.0, 0.0], [0.0, 75.0, 0.0], [0.0, 45.0, 0.0], [0.0, -0.005, 0.017], [-45.0, 45.0, 0.0], [-45.0, 45.0, 0.0], [45.0, -45.0, 0.0]], "CompNames"=["\"ThumbSphere\"", "\"ThumbMeta\"", "\"ThumbSide\"", "\"ThumbKnuckle\"", "\"ThumbDIP\"", "\"IndexSphere\"", "\"IndexSide\"", "\"IndexKnuckle\"", "\"IndexPIP\"", "\"IndexDIP\"", "\"MiddleSphere\"", "\"MiddleKnuckle\"", "\"MiddlePIP\"", "\"MiddleDIP\"", "\"RingSphere\"", "\"RingSide\"", "\"RingKnuckle\"", "\"RingPIP\"", "\"RingDIP\"", "\"LittleSphere\"", "\"LittleSide\"", "\"LittleKnuckle\"", "\"LittlePIP\"", "\"LittleDIP\"", "\"WristSphere\"", "\"WristRoll\"", "\"WristPitch\"", "\"WristYaw\""]}, 7 "SphereArray":dbl[][](array[numeric])=[[0.0, 0.0, 0.0, 0.1, 0.0, 1.0], [0.0, 0.0, 0.0, 0.1, 0.0, 1.0], [0.0, 0.0, 0.0, 0.1, 0.0, 1.0], [0.0, 0.0, 0.0, 0.1, 0.0, 1.0], [0.0, 0.0, 0.0, 0.1, 0.0, 1.0], [0.0, 0.0, 0.0, 0.1, 0.0, 1.0]] min=-1.0 max=1.0, 9 "Mode":enum16{"Initialize", "Run"}(ring)) -> (0 "CompVals":sgl[][](array[numeric])=[[0.033882782, -0.095822535, -0.025582606], [0.062592156, 0.062592156, 0.062592156], [255.0, 0.0, 0.0], [1.0, 0.0, 0.0], [0.023552487, -0.12300678, -0.0648606], [0.12795074, 0.12795074, 0.12795074], [255.0, 0.0, 0.0], [1.0, 0.0, 0.0], [-0.00053903175, -0.05544679, -0.060918946], [0.13765314, 0.13765314, 0.13765314], [255.0, 0.0, 0.0], [1.0, 0.0, 0.0], [-0.022295069, -0.12304468, -0.06273636], [0.13108887, 0.13108887, 0.13108887], [255.0, 0.0, 0.0], [1.0, 0.0, 0.0], [-0.04409924, -0.098918796, -0.06464548], [0.12684087, 0.12684087, 0.12684087], [255.0, 0.0, 0.0], [1.0, 0.0, 0.0], [-0.020700976, -0.12030596, -0.0269013], [0.080926314, 0.080926314, 0.080926314], [255.0, 0.0, 0.0], [1.0, 0.0, 0.0]], 1 "FNums":i16[](array[numeric])=[8, 10, 11, 13, 8, 10, 11, 13, 8, 10, 11, 13, 8, 10, 11, 13, 8, 10, 11, 13, 8, 10, 11, 13], 3 "CompIdxs":i32[](array[numeric])=[34, 69, 69, 69, 2, 37, 37, 37, 3, 38, 38, 38, 4, 39, 39, 39, 0, 35, 35, 35, 1, 36, 36, 36])   [LabVIEW 2020]
uses:
  <vilib>/imath/engines/lvmath/Plug In/_Char/NIMS_CH_character datatype.ctl
  <vilib>/imath/engines/lvmath/Plug In/_Char/NIMS_CH_String to Character Array.vi
  <vilib>/imath/engines/lvmath2/RunTimeEngine/BuiltInFunctions/length/NIMS_length(GV).vi
  <instcachedir>/0/NIMS_length(GV)_08A3D13377FD4E4B96F5795FBF3698FA.lvgen/NIMS_length(GV)_08A3D13377FD4E4B96F5795FBF3698FA_000.vi
  <vilib>/imath/engines/lvmath2/RunTimeEngine/BuiltInFunctions/zeros/NIMS_M=zeros(I32,I32).vi
  <vilib>/imathl/engines/lvmath/Functions/Error Handling/Create Error.vi
  <vilib>/imath/engines/lvmath2/RunTimeEngine/RangeToken/NIMS_Range_R2 - Integer.vi
  <instcachedir>/0/NIMS_Range_R2 - Integer_FFC1A4B1B9F04947ABCB56F009996D55.lvgen/NIMS_Range_R2 - Integer_FFC1A4B1B9F04947ABCB56F009996D55_000.vi
  <vilib>/imath/engines/lvmath2/RunTimeEngine/CommandStatement/MC_CommandStatement_break.vi
  <vilib>/imath/engines/lvmath2/RunTimeSupport/NIMS_Compare Aggregates.vi
  <instcachedir>/0/NIMS_Compare Aggregates_261C0F6E5BD9419EACCA9EC9DF0F8471.lvgen/NIMS_Compare Aggregates_261C0F6E5BD9419EACCA9EC9DF0F8471_000.vi
  <vilib>/imath/engines/lvmath2/RunTimeEngine/IndexRead/NIMS M(V,$).vi
  <instcachedir>/0/NIMS M(V,$)_21A5155762F74C04AE4EA67BEE0D3EF5.lvgen/NIMS M(V,$)_21A5155762F74C04AE4EA67BEE0D3EF5_004.vi
  <vilib>/imath/engines/lvmath2/RunTimeEngine/IndexRead/NIMS V(S).vi
  <instcachedir>/0/NIMS V(S)_0488751826AF41519A22953C041130DC.lvgen/NIMS V(S)_0488751826AF41519A22953C041130DC_000.vi
  <vilib>/imath/engines/lvmath2/RunTimeEngine/ErrorHandling/NIMS_Create Error From Enums.vi
  Documents/LabVIEW Data/MathScriptVIs/MCStatic_53690370032_00c3b45d1a4005535b4c7155b1694066.vi
  <instcachedir>/0/MCStatic_53690370032_00c3b45d1a4005535b4c7155b1694066_C3BDE9DD2420425DA86ABBC8B9DD4E20.lvgen/MCStatic_53690370032_00c3b45d1a4005535b4c7155b1694066_C3BDE9DD2420425DA86ABBC8B9DD4E20_000.vi
  <vilib>/imath/engines/lvmath2/RunTimeEngine/IndexRead/NIMS M(S,$).vi
  <instcachedir>/0/NIMS M(S,$)_F24F360562DE41D8BE234322A2E15C65.lvgen/NIMS M(S,$)_F24F360562DE41D8BE234322A2E15C65_000.vi
  <instcachedir>/0/MCStatic_53690370032_00c3b45d1a4005535b4c7155b1694066_C3BDE9DD2420425DA86ABBC8B9DD4E20.lvgen/MCStatic_53690370032_00c3b45d1a4005535b4c7155b1694066_C3BDE9DD2420425DA86ABBC8B9DD4E20_001.vi
  <instcachedir>/0/MCStatic_53690370032_00c3b45d1a4005535b4c7155b1694066_C3BDE9DD2420425DA86ABBC8B9DD4E20.lvgen/MCStatic_53690370032_00c3b45d1a4005535b4c7155b1694066_C3BDE9DD2420425DA86ABBC8B9DD4E20_002.vi
  <vilib>/imath/engines/lvmath2/RunTimeEngine/VariableToken/NIMS_VariableToken_CondDefined.vi
  <instcachedir>/0/NIMS_VariableToken_CondDefined_537E119D71C74F9D9452D6FF923F1E1F.lvgen/NIMS_VariableToken_CondDefined_537E119D71C74F9D9452D6FF923F1E1F_003.vi
  <vilib>/imath/engines/lvmath2/RunTimeEngine/IndexRead/NIMS V(R2).vi
  <instcachedir>/0/NIMS V(R2)_C76619605A0E4E9F8B2FA9389712AC47.lvgen/NIMS V(R2)_C76619605A0E4E9F8B2FA9389712AC47_000.vi
  <vilib>/imath/engines/lvmath2/RunTimeEngine/IndexRead/NIMS M(R2,$).vi
  <instcachedir>/0/NIMS M(R2,$)_AD8DC2FC79024024B2717E13B4A0EB4B.lvgen/NIMS M(R2,$)_AD8DC2FC79024024B2717E13B4A0EB4B_000.vi
  Documents/LabVIEW Data/MathScriptVIs/MCStatic_53690370032_bbf07314f1ebc27f05637bf870f0e796.vi
  <instcachedir>/0/MCStatic_53690370032_bbf07314f1ebc27f05637bf870f0e796_774DEB751A5C42B29DA90DEEBC4B297E.lvgen/MCStatic_53690370032_bbf07314f1ebc27f05637bf870f0e796_774DEB751A5C42B29DA90DEEBC4B297E_000.vi
  <vilib>/imath/engines/lvmath2/RunTimeEngine/IndexReplace/NIMS M($,S)=V.vi
  <instcachedir>/0/NIMS M($,S)=V_85A28EB895514E96A13A10261726EE3A.lvgen/NIMS M($,S)=V_85A28EB895514E96A13A10261726EE3A_001.vi
  <vilib>/imath/engines/lvmath2/RunTimeEngine/BuiltInFunctions/difference/NIMS_difference(GM,I32).vi
  <instcachedir>/0/NIMS_difference(GM,I32)_0CE67306147646B5B8BCC932BE58DF56.lvgen/NIMS_difference(GM,I32)_0CE67306147646B5B8BCC932BE58DF56_000.vi
  <vilib>/imath/engines/lvmath2/RunTimeEngine/BuiltInFunctions/sum/NIMS_sum(GM,Sca).vi
  <instcachedir>/0/NIMS_sum(GM,Sca)_BFF867FCA20B40888962313BF0DBA2C0.lvgen/NIMS_sum(GM,Sca)_BFF867FCA20B40888962313BF0DBA2C0_001.vi
  <vilib>/imath/engines/lvmath2/RunTimeEngine/BuiltInFunctions/sum/NIMS_sum(GV).vi
  <instcachedir>/0/NIMS_sum(GV)_67F5EC36BC034E54A6BEC5B0673C00E5.lvgen/NIMS_sum(GV)_67F5EC36BC034E54A6BEC5B0673C00E5_001.vi
  <vilib>/imath/engines/lvmath2/RunTimeEngine/NodeEndStatement/NIMS_NodeEndStatement_Output.vi
  <instcachedir>/0/NIMS_NodeEndStatement_Output_53EC0D466D134D7ABD903AC30B43404B.lvgen/NIMS_NodeEndStatement_Output_53EC0D466D134D7ABD903AC30B43404B_001.vi
  <vilib>/imath/engines/lvmath2/RunTimeEngine/ErrorHandling/NIMS_Finalize Error.vi
  <instcachedir>/0/NIMS_NodeEndStatement_Output_53EC0D466D134D7ABD903AC30B43404B.lvgen/NIMS_NodeEndStatement_Output_53EC0D466D134D7ABD903AC30B43404B_005.vi
  FeedbackDecode_calcXYZ.m
  FeedbackDecode_interpCompBnds.m
panel:
  out "MType":i16
  in  "SpherePosCluster":T3(array[cluster])=[{"Name"="ThumbSpherePos", "CompIdxs"=[34, 69, 12, 32, 20, 14, 65], "CompBnds"=[[nan, nan], [nan, nan], [0.0, 45.0], [-40.0, 40.0], [-25.0, 25.0], [0.0, 75.0], [nan, nan]], "ComCOM"=[[0.0, 0.0, 0.0], [0.0, 0.0, 0.0], [0.021492499999999998, -0.03378899999999996, -0.00419606], [0.02109500000000001, 0.004157999999999995, 0.0011177799999999996], [0.02141599999999999, -0.02498200000000006, -0.019637099999999998], [-0.0038744, -0.03277199999999991, -0.00013860000000000088], [0.000247200000000003, -0.009821999999999997, 0.002948000000000001]], "CompRot"=[[0.0, 0.0, 0.0], [0.0, 0.0, 0.0], [-0.0535837, 0.998379, -0.01917], [-0.996987, -0.0545675, -0.0551262], [0.0553349, -0.00232049, -0.998465], [0.0553349, -0.00232049, -0.998465], [0.0, 0.0, 0.0]], "Offset"=[-0.01, -0.0075, 0.0], "FNums"=[8, 10, 11, 13], "ArcLength"=0.0312960774439215, "CompNames"=[["\"ThumbSphereJ\"", "\"ThumbSphereJ\""], ["\"ThumbSphere\"", "\"ThumbSphere\""], ["\"ThumbMeta\"", "\"ThumbMeta\""], ["\"ThumbSide\"", "\"ThumbSide\""], ["\"ThumbKnuckle\"", "\"ThumbKnuckle\""], ["\"ThumbDIP\"", "\"ThumbDIP\""], ["\"ThumbDistal\"", "\"ThumbDistal\""]]}, {"Name"="IndexSpherePos", "CompIdxs"=[2, 37, 19, 26, 28, 8, 57], "CompBnds"=[[nan, nan], [nan, nan], [10.0, -13.0], [0.0, 75.0], [0.0, 75.0], [0.0, 45.0], [nan, nan]], "ComCOM"=[[0.0, 0.0, 0.0], [0.0, 0.0, 0.0], [0.021764900000000004, -0.07256200000000002, 0.009436320000000002], [-0.0022342000000000056, -0.01748099999999997, -0.01128254], [-0.0025014999999999968, -0.04095799999999994, 0.00216769], [0.0004009999999999986, -0.025998999999999994, -0.00022586999999999954], [0.006452400000000004, -0.010254000000000096, 0.00201137]], "CompRot"=[[0.0, 0.0, 0.0], [0.0, 0.0, 0.0], [-0.0293463, 0.0474512, -0.998442], [0.999568, -9.94013e-05, -0.0293841], [0.999568, -9.94013e-05, -0.0293841], [0.999568, -9.94013e-05, -0.0293841], [0.0, 0.0, 0.0]], "Offset"=[0.0, -0.005, -0.0075], "FNums"=[8, 10, 11, 13], "ArcLength"=0.06397537430118536, "CompNames"=[["\"IndexSphereJ\"", "\"IndexSphereJ\""], ["\"IndexSphere\"", "\"IndexSphere\""], ["\"IndexSide\"", "\"IndexSide\""], ["\"IndexKnuckle\"", "\"IndexKnuckle\""], ["\"IndexPIP\"", "\"IndexPIP\""], ["\"IndexDIP\"", "\"IndexDIP\""], ["\"IndexDistal\"", "\"IndexDistal\""]]}, {"Name"="MiddleSpherePos", "CompIdxs"=[3, 38, 33, 22, 6, 62], "CompBnds"=[[nan, nan], [nan, nan], [0.0, 75.0], [0.0, 75.0], [0.0, 45.0], [nan, nan]], "ComCOM"=[[0.0, 0.0, 0.0], [0.0, 0.0, 0.0], [-0.0022194, -0.01828099999999999, 0.00887662], [-0.0053969, -0.047905000000000086, -0.0012990999999999992], [-4.380000000000009e-05, -0.02600199999999997, -0.00032900000000000117], [0.006214500000000001, -0.010195999999999983, 0.002865300000000001]], "CompRot"=[[0.0, 0.0, 0.0], [0.0, 0.0, 0.0], [0.999848, -0.0174524, 0.0], [0.999848, -0.0174524, 0.0], [0.999848, -0.0174524, 0.0], [0.0, 0.0, 0.0]], "Offset"=[0.0, -0.005, -0.0075], "FNums"=[8, 10, 11, 13], "ArcLength"=0.0688265730936801, "CompNames"=[["\"MiddleSphereJ\"", "\"MiddleSphereJ\""], ["\"MiddleSphere\"", "\"MiddleSphere\""], ["\"MiddleKnuckle\"", "\"MiddleKnuckle\""], ["\"MiddlePIP\"", "\"MiddlePIP\""], ["\"MiddleDIP\"", "\"MiddleDIP\""], ["\"MiddleDistal\"", "\"MiddleDistal\""]]}, {"Name"="RingSpherePos", "CompIdxs"=[4, 39, 7, 9, 21, 13, 46], "CompBnds"=[[nan, nan], [nan, nan], [-10.0, 10.0], [0.0, 75.0], [0.0, 75.0], [0.0, 45.0], [nan, nan]], "ComCOM"=[[0.0, 0.0, 0.0], [0.0, 0.0, 0.0], [-0.02101538, -0.07147700000000001, 0.011873520000000002], [-0.0044852699999999995, -0.01782399999999995, -0.01056839], [-0.00383984, -0.04091100000000003, 0.0002926500000000002], [-0.0004015900000000003, -0.02599600000000002, 0.00045404999999999925], [0.0060837420000000005, -0.01019099999999995, 0.003152490000000001]], "CompRot"=[[0.0, 0.0, 0.0], [0.0, 0.0, 0.0], [-0.00232535, 0.00435695, -0.999988], [0.999508, -0.0312549, -0.00246041], [0.999508, -0.0312549, -0.00246041], [0.999508, -0.0312549, -0.00246041], [0.0, 0.0, 0.0]], "Offset"=[0.0, -0.005, -0.0075], "FNums"=[8, 10, 11, 13], "ArcLength"=0.0655444335097331, "CompNames"=[["\"RingSphereJ\"", "\"RingSphereJ\""], ["\"RingSphere\"", "\"RingSphere\""], ["\"RingSide\"", "\"RingSide\""], ["\"RingKnuckle\"", "\"RingKnuckle\""], ["\"RingPIP\"", "\"RingPIP\""], ["\"RingDIP\"", "\"RingDIP\""], ["\"RingDistal\"", "\"RingDistal\""]]}, {"Name"="LittleSpherePos", "CompIdxs"=[0, 35, 11, 23, 18, 25, 49], "CompBnds"=[[nan, nan], [nan, nan], [-8.0, 15.0], [0.0, 75.0], [0.0, 75.0], [0.0, 45.0], [nan, nan]], "ComCOM"=[[0.0, 0.0, 0.0], [0.0, 0.0, 0.0], [-0.041231000000000004, -0.04929499999999998, 0.0061943200000000006], [-0.004357399999999997, -0.01773199999999997, -0.01077354], [-0.0041499000000000015, -0.03644100000000006, 0.0013829099999999998], [-0.0007269999999999985, -0.025963999999999987, 0.00124127], [0.005866699999999999, -0.010155000000000025, 0.003641860000000001]], "CompRot"=[[0.0, 0.0, 0.0], [0.0, 0.0, 0.0], [0.0282614, 0.00816239, -0.999567], [0.99871, -0.0424232, 0.0278908], [0.99871, -0.0424232, 0.0278908], [0.99871, -0.0424232, 0.0278908], [0.0, 0.0, 0.0]], "Offset"=[0.0, -0.005, -0.0075], "FNums"=[8, 10, 11, 13], "ArcLength"=0.06342043485566709, "CompNames"=[["\"LittleSphereJ\"", "\"LittleSphereJ\""], ["\"LittleSphere\"", "\"LittleSphere\""], ["\"LittleSide\"", "\"LittleSide\""], ["\"LittleKnuckle\"", "\"LittleKnuckle\""], ["\"LittlePIP\"", "\"LittlePIP\""], ["\"LittleDIP\"", "\"LittleDIP\""], ["\"LittleDistal\"", "\"LittleDistal\""]]}, {"Name"="WristSpherePos", "CompIdxs"=[1, 36, 17, 5, 10, 41], "CompBnds"=[[nan, nan], [nan, nan], [-45.0, 45.0], [45.0, -45.0], [-45.0, 45.0], [nan, nan]], "ComCOM"=[[0.0, 0.0, 0.0], [0.0, 0.0, 0.0], [-0.0007346999999999996, -0.04209300000000005, 0.0], [0.0054991, -9.599999999998499e-05, 0.01685], [0.0028509999999999994, -0.030055000000000054, -0.017305920000000002], [0.0028059999999999995, -0.03790699999999991, -0.0002803999999999992]], "CompRot"=[[0.0, 0.0, 0.0], [0.0, 0.0, 0.0], [0.0174524, 0.999848, 0.0], [0.0, 0.0, -1.0], [0.999848, -0.0174524, 0.0], [0.0, 0.0, 0.0]], "Offset"=[-0.04, -0.01, -0.017], "FNums"=[8, 10, 11, 13], "ArcLength"=0.04046315717886194, "CompNames"=[["\"WristSphereJ\"", "\"WristSphereJ\""], ["\"WristSphere\"", "\"WristSphere\""], ["\"WristRoll\"", "\"WristRoll\""], ["\"WristPitch\"", "\"WristYaw\""], ["\"WristYaw\"", "\"WristPitch\""], ["\"PalmAssembly\"", "\"PalmAssembly\""]]}]
  # "Thumb\nIndex\nMiddle\nRing\nLittle\nWrist"
  # "Position, PositionInt, PositionRoll, Size, Color, Visibility"
  # "CompNames: Index 0 (left hand), Index 1 (right hand)"
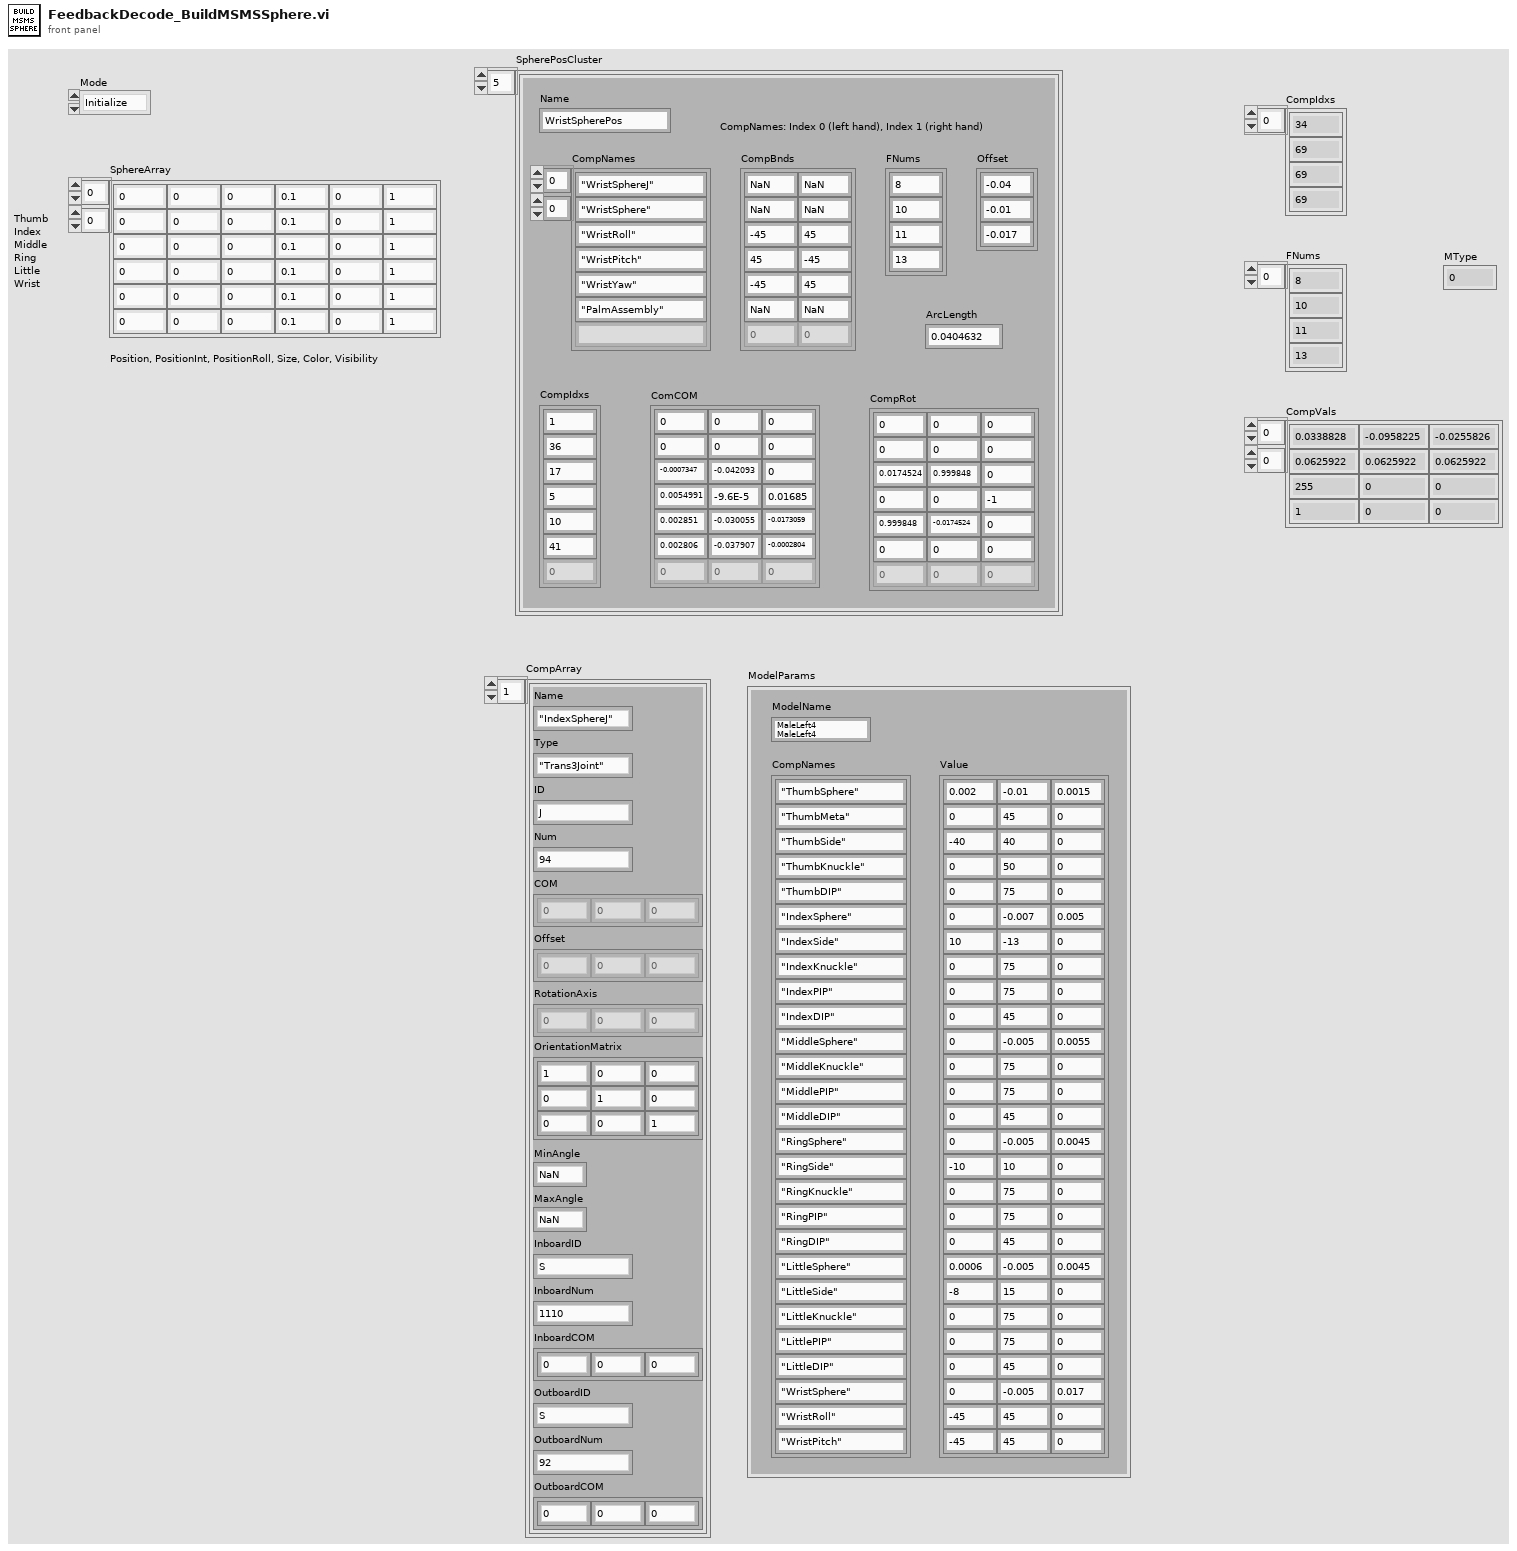
[diagram p1: front panel]
types:
  T1 = cluster{"ModelName":string, "Value":dbl[][], "CompNames":string[]}
  T2 = cluster{"Name":string, "Type":string, "ID":string, "Num":string, "COM":dbl[], "Offset":dbl[], "RotationAxis":dbl[], "OrientationMatrix":dbl[][], "MinAngle":dbl, "MaxAngle":dbl, "InboardID":string, "InboardNum":string, "InboardCOM":dbl[], "OutboardID":string, "OutboardNum":string, "OutboardCOM":dbl[]}[]
  T3 = cluster{"Name":string, "CompIdxs":i32[], "CompBnds":dbl[][], "ComCOM":dbl[][], "CompRot":dbl[][], "Offset":dbl[], "FNums":i16[], "ArcLength":dbl, "CompNames":string[][]}[]
  T4 = typedef "NIMS_CH_character datatype.ctl" = cluster{"Numeric":u8}
  T5 = cluster{"Name":string, "Type":string, "ID":string, "Num":string, "COM":dbl[], "Offset":dbl[], "RotationAxis":dbl[], "OrientationMatrix":dbl[][], "MinAngle":dbl, "MaxAngle":dbl, "InboardID":string, "InboardNum":string, "InboardCOM":dbl[], "OutboardID":string, "OutboardNum":string, "OutboardCOM":dbl[]}
  T6 = cluster{"Name":string, "CompIdxs":i32[], "CompBnds":dbl[][], "ComCOM":dbl[][], "CompRot":dbl[][], "Offset":dbl[], "FNums":i16[], "ArcLength":dbl, "CompNames":string[][]}
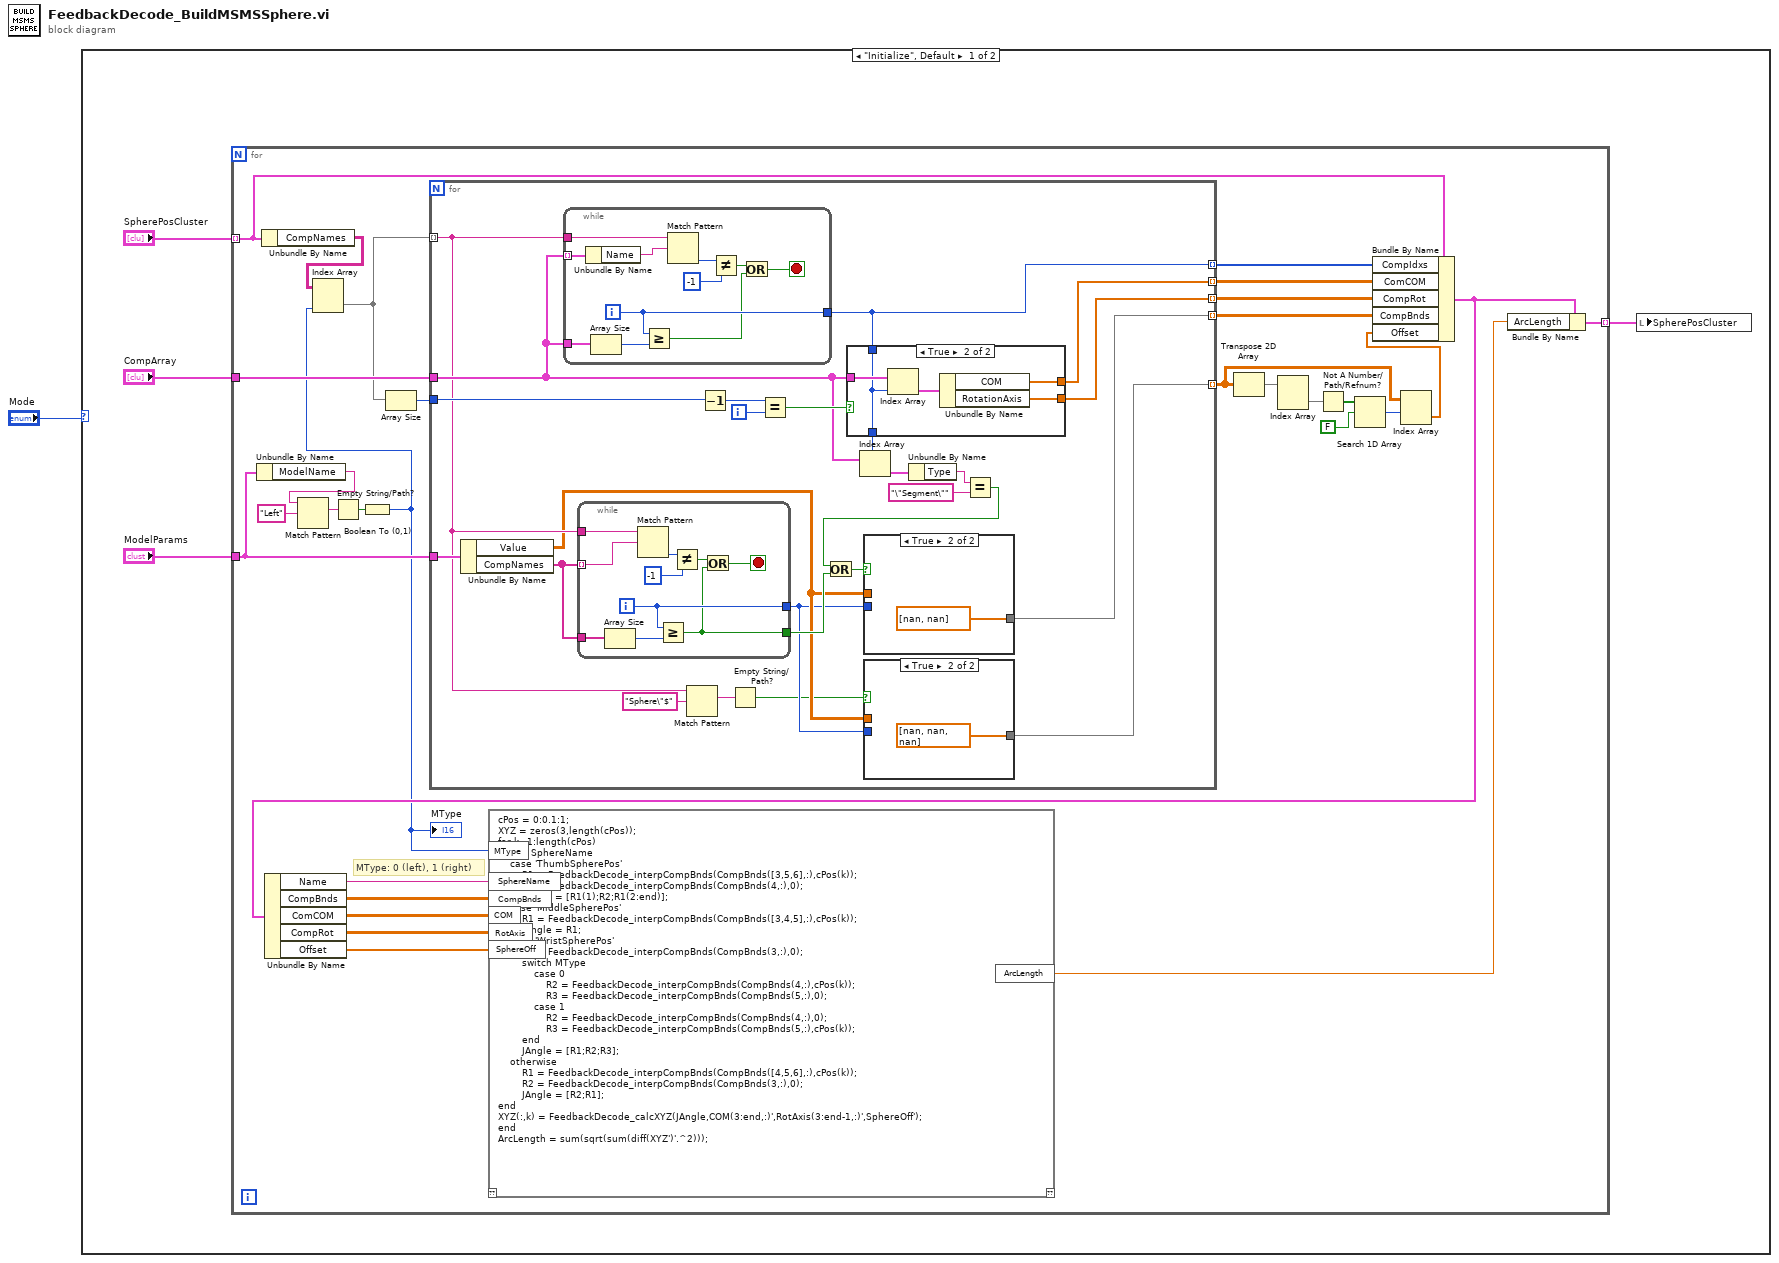
[diagram p0: block diagram]
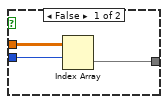
[diagram p2: hidden frame]
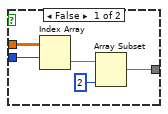
[diagram p3: hidden frame]
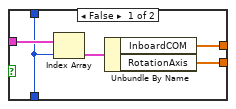
[diagram p4: hidden frame]
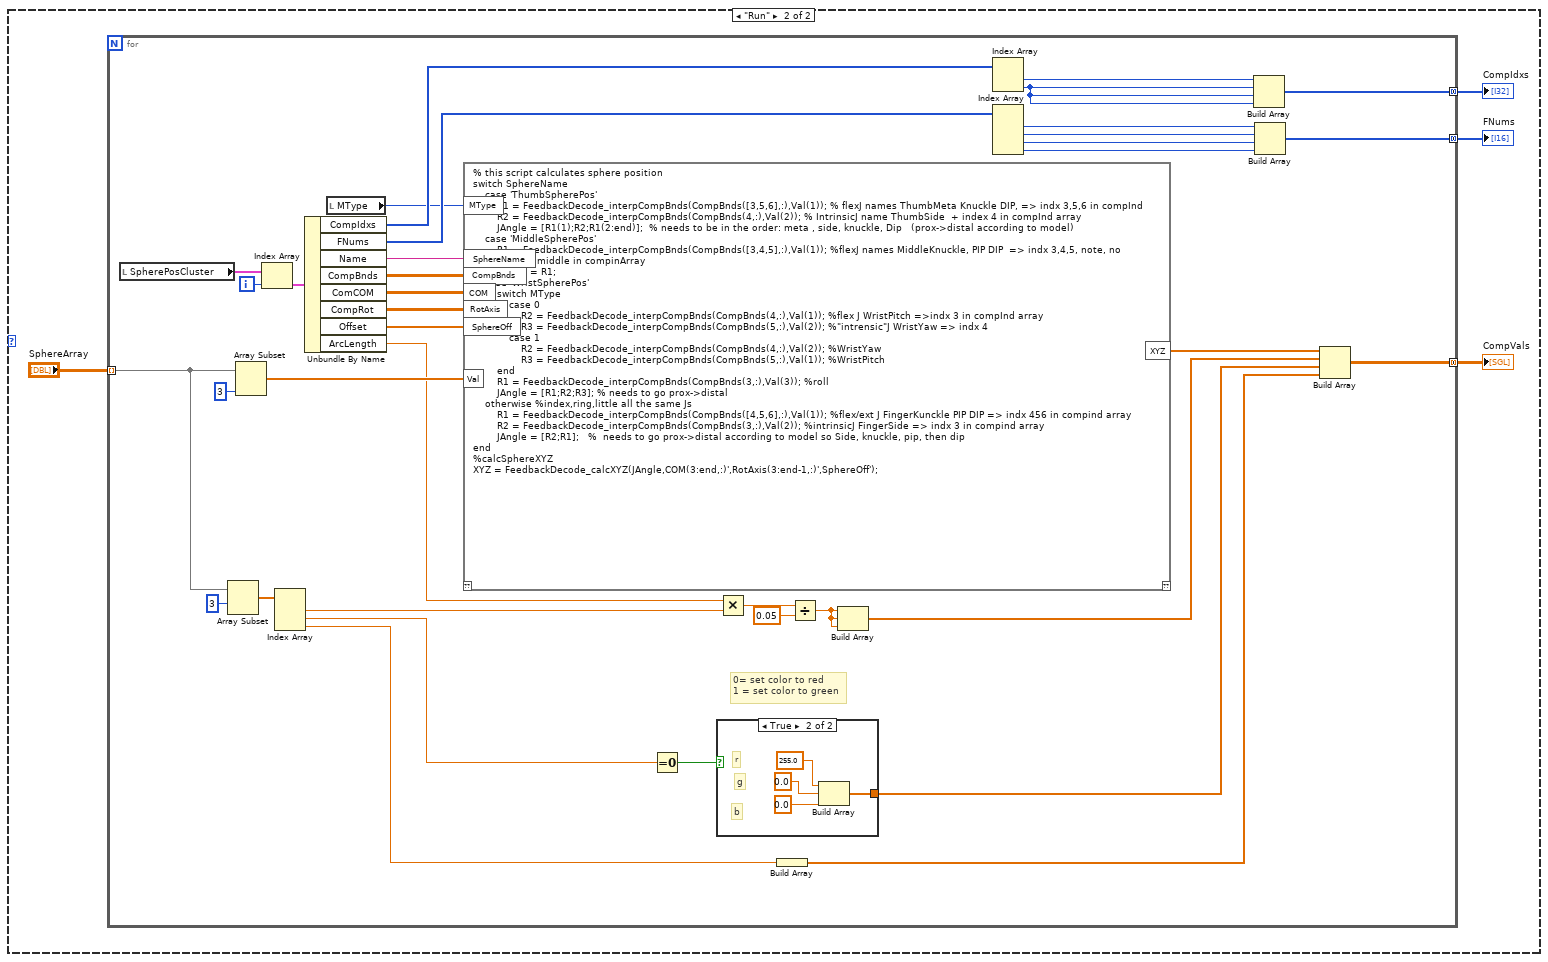
[diagram p5: hidden frame]
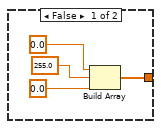
[diagram p6: hidden frame]
diagram:
  n1 = case shown="\"Initialize\", Default" "Mode" {
    frame "Initialize", Default {
      n2 = for {
        tunnel: "SpherePosCluster" -> [w32] mode=indexing
        tunnel: "CompArray" -> [w35]
        tunnel: [w29] -> w5 mode=indexing
        tunnel: "ModelParams" -> [w13]
        # "MType: 0 (left), 1 (right)"
        n3 = Unbundle By Name(w13) -> ("ModelName"=w12:string)
        n4 = Unbundle By Name(w32) -> ("CompNames"=w8:string[][])
        n5 = Match Pattern(string=w12, regular expression="Left") -> (match substring=w10:string)  [unwired: 1 in, 3 out]
        n6 = Empty String/Path?(string/path=w10) -> (empty?=w9:bool)
        n7 = Boolean To (0,1)(Boolean=w9) -> (0, 1=w6:i16)
        "MType" <- w6
        n8 = Index Array(array=w8, index (col)=w6) -> (element=w7:string[])  [unwired: 1 in]
        n9 = Array Size(array=w7) -> (size(s)=w33:i32)
        n10 = for {
          tunnel: w7 -> [w706] mode=indexing
          tunnel: [w724] -> w34 mode=indexing
          tunnel: w35 -> [w714]
          tunnel: [w723] -> w28 mode=indexing
          tunnel: [w722] -> w27 mode=indexing
          tunnel: w33 -> [w721]
          tunnel: w13 -> [w716]
          tunnel: [w707] -> w26 mode=indexing
          tunnel: [w700] -> w21 mode=indexing
          i -> [w718]
          n11 = Unbundle By Name(w716) -> ("Value"=w704:dbl[][], "CompNames"=w717:string[])
          n12 = while {
            tunnel: w706 -> [w765]
            tunnel: w714 -> [w764] mode=indexing
            tunnel: [w758] -> w724
            tunnel: w714 -> [w760]
            i -> [w758]
            stop <- w755 stop-if-true
            n13 = Unbundle By Name(w764) -> ("Name"=w763:string)
            n14 = Array Size(array=w760) -> (size(s)=w759:i32)
            n15 = Greater Or Equal?(x=w758, y=w759) -> (x >= y?=w756:bool)
            n16 = Match Pattern(string=w765, regular expression=w763) -> (offset past match=w761:i32)  [unwired: 1 in, 3 out]
            n17 = Not Equal?(x=w761, y=-1) -> (x != y?=w757:bool)
            n18 = Or(x=w757, y=w756) -> (x .or. y?=w755:bool)
          }
          n19 = while {
            tunnel: w706 -> [w744]
            tunnel: w717 -> [w737]
            tunnel: w717 -> [w738] mode=indexing
            tunnel: [w736] -> w703
            tunnel: [w735] -> w709
            i -> [w736]
            stop <- w739 stop-if-true
            n20 = Array Size(array=w737) -> (size(s)=w741:i32)
            n21 = Match Pattern(string=w744, regular expression=w738) -> (offset past match=w742:i32)  [unwired: 1 in, 3 out]
            n22 = Greater Or Equal?(x=w736, y=w741) -> (x >= y?=w735:bool)
            n23 = Not Equal?(x=w742, y=-1) -> (x != y?=w740:bool)
            n24 = Or(x=w740, y=w735) -> (x .or. y?=w739:bool)
          }
          n25 = Match Pattern(string=w706, regular expression="Sphere\"$") -> (match substring=w702:string)  [unwired: 1 in, 3 out]
          n26 = Decrement(x=w721) -> (x-1=w720:i32)
          n27 = Empty String/Path?(string/path=w702) -> (empty?=w701:bool)
          n28 = Equal?(x=w720, y=w718) -> (x = y?=w719:bool)
          n29 = case shown="True" w719 {
            tunnel: w714 -> [w749 w753]
            tunnel: w724 -> [w745 w750]
            tunnel: [w747 w752] -> w723
            tunnel: [w746 w751] -> w722
            tunnel: [w745 w750] -> w715
            frame False {
              n30 = Index Array(array=w749, index=w745) -> (element=w748:T5)
              n31 = Unbundle By Name(w748) -> ("InboardCOM"=w747:dbl[], "RotationAxis"=w746:dbl[])
            }
            frame True {
              n32 = Index Array(array=w753, index=w750) -> (element=w754:T5)
              n33 = Unbundle By Name(w754) -> ("COM"=w752:dbl[], "RotationAxis"=w751:dbl[])
            }
          }
          n34 = Index Array(array=w714, index=w715) -> (element=w713:T5)
          n35 = case shown="True" w701 {
            tunnel: w704 -> [w727 _]
            tunnel: w703 -> [w726 _]
            tunnel: [w725 dbl[] [nan, nan, nan] ("subarray")] -> w700
            frame False {
              n36 = Index Array(array=w727, index (row)=w726) -> (element=w725:dbl[])  [unwired: 1 in]
            }
            frame True {
            }
          }
          n37 = Unbundle By Name(w713) -> ("Type"=w712:string)
          n38 = Equal?(x=w712, y="\"Segment\"") -> (x = y?=w708:bool)
          n39 = Or(x=w708, y=w709) -> (x .or. y?=w710:bool)
          n40 = case shown="True" w710 {
            tunnel: w704 -> [w731 _]
            tunnel: w703 -> [w730 _]
            tunnel: [w729 dbl[] [nan, nan] ("subarray")] -> w707
            frame False {
              n41 = Index Array(array=w731, index (row)=w730) -> (element=w732:dbl[])  [unwired: 1 in]
              n42 = Array Subset(array=w732, length=2) -> (w729:dbl[])  [unwired: 1 in]
            }
            frame True {
            }
          }
        }
        n43 = Transpose 2D Array(2D array=w21) -> (transposed array=w24:dbl[][])
        n44 = Index Array(array=w24) -> (element=w23:dbl[])  [unwired: 2 in]
        n45 = Not A Number/Path/Refnum?(number/path/refnum=w23) -> (NaN/Path/Refnum?=w25:bool[])
        n46 = Search 1D Array(1D array=w25, element=FALSE) -> (index of element=w22:i32)  [unwired: 1 in]
        n47 = Index Array(array=w21, index (row)=w22) -> (element=w20:dbl[])  [unwired: 1 in]
        n48 = Bundle By Name(cluster=w32, "CompIdxs"=w34, "ComCOM"=w28, "CompRot"=w27, "CompBnds"=w26, "Offset"=w20) -> (w31:T6)
        n49 = Unbundle By Name(w31) -> ("Name"=w18:string, "CompBnds"=w17:dbl[][], "ComCOM"=w16:dbl[][], "CompRot"=w15:dbl[][], "Offset"=w14:dbl[])
        n50 = mathscript code="cPos = 0:0.1:1;\nXYZ = zeros(3,length(cPos));\nfor k=1:length(cPos)\nswitch SphereName\n    case 'ThumbSpherePos'        \n        R1 = FeedbackDecode_interpCompBnds(CompBnds([3,5,6],:),cPos(k)); \n        R2 = FeedbackDecode_interpCompBnds(CompBnds(4,:),0); \n        JAngle = [R1(1);R2;R1(2:end)];  \n    case 'MiddleSpherePos'\n        R1 = FeedbackDecode_interpCompBnds(CompBnds([3,4,5],:),cPos(k)); \n        JAngle = R1;              \n    case 'WristSpherePos'     \n        R1 = FeedbackDecode_interpCompBnds(CompBnds(3,:),0);\n        switch MType\n            case 0\n                R2 = FeedbackDecode_interpCompBnds(CompBnds(4,:),cPos(k)); \n                R3 = FeedbackDecode_interpCompBnds(CompBnds(5,:),0); \n            case 1\n                R2 = FeedbackDecode_interpCompBnds(CompBnds(4,:),0); \n                R3 = FeedbackDecode_interpCompBnds(CompBnds(5,:),cPos(k)); \n        end           \n        JAngle = [R1;R2;R3]; \n    otherwise \n        R1 = FeedbackDecode_interpCompBnds(CompBnds([4,5,6],:),cPos(k)); \n        R2 = FeedbackDecode_interpCompBnds(CompBnds(3,:),0); \n        JAngle = [R2;R1]; \nend\nXYZ(:,k) = FeedbackDecode_calcXYZ(JAngle,COM(3:end,:)',RotAxis(3:end-1,:)',SphereOff');\nend\nArcLength = sum(sqrt(sum(diff(XYZ')'.^2)));"("CompBnds"=w17, "COM"=w16, "RotAxis"=w15, "SphereOff"=w14, "SphereName"=w18, "MType"=w6) -> ("ArcLength"=w30:dbl)  [unwired: 1 in, 1 out]
        n51 = Bundle By Name(cluster=w31, "ArcLength"=w30) -> (w29:T6)
      }
      n52 = local write "SpherePosCluster"(w5) -> ()
    }
    frame "Run" {
      n53 = for {
        tunnel: "SphereArray" -> [w784] mode=indexing
        tunnel: [w792] -> w768 mode=concatenating
        tunnel: [w790] -> w767 mode=concatenating
        tunnel: [w787] -> w766 mode=concatenating
        i -> [w805]
        # "0= set color to red \n1 = set color to green"
        n54 = local read "SpherePosCluster"() -> (w804:T3)
        n55 = Array Subset(array=w784, index=3) -> (w797:dbl[])  [unwired: 1 in]
        n56 = Array Subset(array=w784, length=3) -> (w799:dbl[])  [unwired: 1 in]
        n57 = Index Array(array=w804, index=w805) -> (element=w806:T6)
        n58 = Index Array(array=w797) -> (element #1=w779:dbl, element #2=w781:dbl, element #3=w774:dbl)  [unwired: 3 in]
        n59 = Unbundle By Name(w806) -> ("CompIdxs"=w801:i32[], "FNums"=w793:i16[], "Name"=w796:string, "CompBnds"=w795:dbl[][], "ComCOM"=w794:dbl[][], "CompRot"=w803:dbl[][], "Offset"=w802:dbl[], "ArcLength"=w780:dbl)
        n60 = local read "MType"() -> (w770:i16)
        n61 = mathscript code="% this script calculates sphere position\nswitch SphereName\n    case 'ThumbSpherePos'        \n        R1 = FeedbackDecode_interpCompBnds(CompBnds([3,5,6],:),Val(1)); % flexJ names ThumbMeta Knuckle DIP, => indx 3,5,6 in compInd\n        R2 = FeedbackDecode_interpCompBnds(CompBnds(4,:),Val(2)); % IntrinsicJ name ThumbSide  + index 4 in compInd array\n        JAngle = [R1(1);R2;R1(2:end)];  % needs to be in the order: meta , side, knuckle, Dip   (prox->distal according to model)                     \n    case 'MiddleSpherePos'\n        R1 = FeedbackDecode_interpCompBnds(CompBnds([3,4,5],:),Val(1)); %flexJ names MiddleKnuckle, PIP DIP  => indx 3,4,5, note, no intrensicJ for middle in compinArray     \n        JAngle = R1;              \n    case 'WristSpherePos'\n        switch MType\n            case 0\n                R2 = FeedbackDecode_interpCompBnds(CompBnds(4,:),Val(1)); %flex J WristPitch =>indx 3 in compInd array\n                R3 = FeedbackDecode_interpCompBnds(CompBnds(5,:),Val(2)); %\"intrensic\"J WristYaw => indx 4\n            case 1\n                R2 = FeedbackDecode_interpCompBnds(CompBnds(4,:),Val(2)); %WristYaw\n                R3 = FeedbackDecode_interpCompBnds(CompBnds(5,:),Val(1)); %WristPitch\n        end\n        R1 = FeedbackDecode_interpCompBnds(CompBnds(3,:),Val(3)); %roll               \n        JAngle = [R1;R2;R3]; % needs to go prox->distal\n    otherwise %index,ring,little all the same Js\n        R1 = FeedbackDecode_interpCompBnds(CompBnds([4,5,6],:),Val(1)); %flex/ext J FingerKunckle PIP DIP => indx 456 in compind array\n        R2 = FeedbackDecode_interpCompBnds(CompBnds(3,:),Val(2)); %intrinsicJ FingerSide => indx 3 in compind array\n        JAngle = [R2;R1];   %  needs to go prox->distal according to model so Side, knuckle, pip, then dip              \nend\n%calcSphereXYZ\nXYZ = FeedbackDecode_calcXYZ(JAngle,COM(3:end,:)',RotAxis(3:end-1,:)',SphereOff');"("CompBnds"=w795, "Val"=w799, "COM"=w794, "RotAxis"=w803, "SphereOff"=w802, "SphereName"=w796, "MType"=w770) -> ("XYZ"=w789:dbl[])  [unwired: 1 in, 1 out]
        n62 = Equal To 0?(x=w781) -> (x = 0?=w785:bool)
        n63 = case shown="True" w785 {
          tunnel: [w807 w814] -> w782
          frame False {
            n64 = Build Array(0.0, 255.0, 0.0) -> (w807:dbl[])
          }
          frame True {
            # "b"
            # "g"
            # "r"
            n65 = Build Array(255.0, 0.0, 0.0) -> (w814:dbl[])
          }
        }
        n66 = Multiply(x=w780, y=w779) -> (x*y=w778:dbl)
        n67 = Build Array(w774) -> (w773:dbl[])
        n68 = Divide(x=w778, y=0.05) -> (x/y=w775:dbl)
        n69 = Build Array(w775, w775, w775) -> (w776:dbl[])
        n70 = Index Array(array=w801) -> (element #1=w786:i32, element #2=w772:i32)  [unwired: 2 in]
        n71 = Index Array(array=w793) -> (element #1=w791:i16, element #2=w788:i16, element #3=w783:i16, element #4=w771:i16)  [unwired: 4 in]
        n72 = Build Array(w786, w772, w772, w772) -> (w792:i32[])
        n73 = Build Array(w791, w788, w783, w771) -> (w790:i16[])
        n74 = Build Array(w789, w776, w782, w773) -> (w787:dbl[][])
      }
      "CompVals" <- w766
      "CompIdxs" <- w768
      "FNums" <- w767
    }
  }
